vi "Initialize Gyro.vi"   [LabVIEW 2018]
uses:
  gyro sensor adis/ADIS16448 IMU/ADIS16448_IMU.lvlib
types:
  T1 = typedef "ADIS16448_IMU.lvlib/ADI_IMU_ADIS16448_IMUDevRef.ctl" = cluster{"DevStatus":errorcluster, "Handle":i32, "SPI Bus":T2, "Device Found":bool, "Device Ready":bool, "Yaw Axis":enum16{"X", "Y", "Z"}, "AHRS Algorithm":enum16{"Complementary", "Madgwick"}, "Serial":u16, "Lot ID 2":u16, "Lot ID 1":u16, "Bytes Per Sample":u16, "Calibrate On Open?":bool}
  T2 = typedef "spi_bus.ctl" = enum16{"SPI On-Board, CS0", "SPI On-Board, CS1", "SPI On-Board, CS2", "SPI On-Board, CS3", "SPI MXP", "Invalid"}
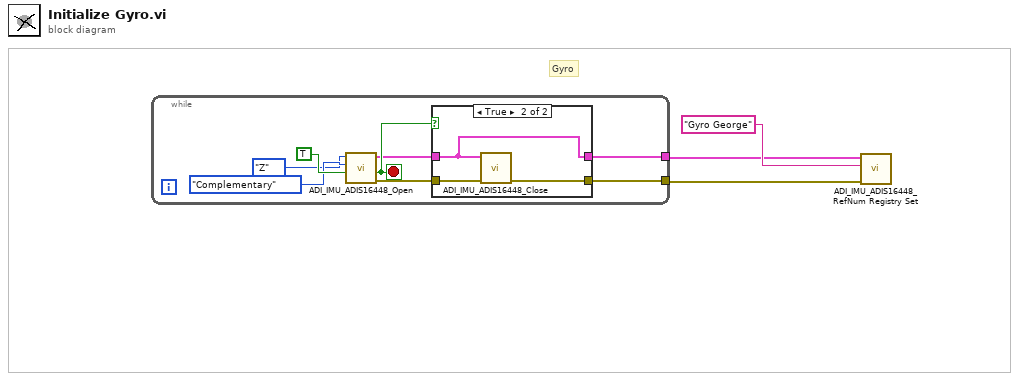
[diagram p0: block diagram]
diagram:
  # "Gyro"
  n1 = while {
    tunnel: [w4] -> w1
    tunnel: [w5] -> w2
    stop <- w8 stop-if-true
    n2 = call "ADI_IMU_ADIS16448_Open.vi"("Calibrate On Open 2"=TRUE ("Calibrate On Open"), "AHRS Algorithm 2"=enum16{"Complementary", "Madgwick"}."Complementary" ("AHRS Algorithm"), "Yaw Axis 2"=enum16{"X", "Y", "Z"}."Z" ("Yaw Axis")) -> ("error out 2"=w6:errorcluster, "error?"=w8:bool, "ADI IMU DevRef Out 2"=w7:T1)  [unwired: 6 in]
    n3 = case shown="True" w8 {
      tunnel: w7 -> [w13 w14]
      tunnel: w6 -> [w12 w16]
      tunnel: [w13 w14] -> w5
      tunnel: [w12 w15] -> w4
      frame False {
      }
      frame True {
        n4 = call "ADI_IMU_ADIS16448_Close.vi"("error in"=w16, "ADI IMU DevRef"=w14) -> ("error out"=w15:errorcluster)  [unwired: 9 in]
      }
    }
  }
  n5 = call "ADI_IMU_ADIS16448_RefNum Registry Set.vi"("error in (no error)"=w1, "refnum name"="Gyro George", "ADI IMU DevRef"=w2) -> ()  [unwired: 7 in, 2 out]
